vi "Read Reporting period.vi"(8 "error in (no error)":errorcluster, 11 "C37.118 Sim in":refnum<class "C37.118 Sim.lvclass">) -> (0 "error out":errorcluster, 2 "Reporting period":dbl, 3 "C37.118 Sim out":refnum<class "C37.118 Sim.lvclass">)   [LabVIEW 2014, in "SensorPlugins.lvlib" / "C37.118 Sim.lvclass"]
uses:
  C37.118 Sim.lvclass
  C37.118 Sim.lvclass/C37.118 Sim.ctl
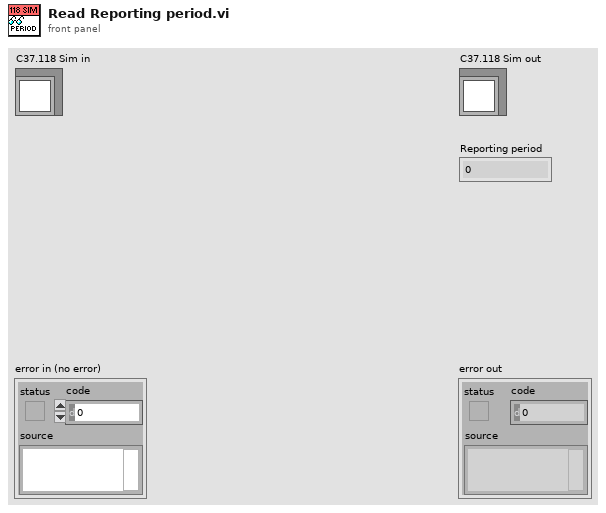
[diagram p1: front panel]
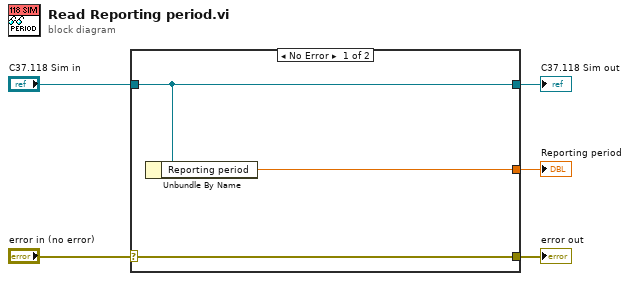
[diagram p0: block diagram]
diagram:
  n1 = case shown="No Error" "error in (no error)" {
    selector: "error in (no error)" -> [w8 w9]
    tunnel: [w8 w9] -> w4
    tunnel: [w7 w10] -> w2
    tunnel: "C37.118 Sim in" -> [w7 w10]
    tunnel: [w6 _] -> w1
    frame No Error {
      n2 = Unbundle By Name(w7) -> ("Reporting period"=w6:dbl)
    }
    frame Error {
    }
  }
  "error out" <- w4
  "C37.118 Sim out" <- w2
  "Reporting period" <- w1
